vi "FR Make Default FRmeter settings.vi"() -> (3 "FFmeter settings":T1={"AC Source"={"AC Source type"=enum."Fluke 5XXX calibrator", "VISA"="", "Ref. clock (Hz)"=0.0, "status ref"=refnum}, "TWM pipe"="\\\\.\\pipe\\TWM:server", "Measurement status ref"=refnum, "TWM Status ref"=refnum, "Abort ref"=refnum, "DC meter"={"DC meter type"=enum."H/A/K 3458", "DC meter VISA"="", "NPLC"=10, "status ref"=refnum}, "Measurement properties"={"Measurement frequencies (Hz)"=[1000.0], "Sampling frequency (Hz)"=500000.0, "Signal amplitude (V)"=4.5, "AC-DC settle time (s)"=20.0, "Record length (multiples of period)"=[1000.0, 10000.0, 1000.0], "Measurement template file"=path "", "Row of START keyword"=1, "Row of STOP keyword"=0, "Calculate RMS from samples"=FALSE, "AC-DC warm up time (s)"=300.0, "Measurement template line"=[], "DC meter readings No."=10, "Algorithm"="TWM-WFFT", "Simultaneous measurement"=FALSE}, "Skip waiting ref"=refnum, "Octave paths"={"GNU Octave path"=path "C:/Program Files/GNU Octave/Octave-6.2.0/mingw64/bin", "TWM+QWTB path"=path "C:/Users/labina/Desktop/TWM-1.8.7.0-full/octprog", "lvlib path"=path "D:/martin/WAC/WACsw - github/control_software/Filter function meter/external libraries/GOLPI 0.7.3.1 source distribution LV 20.0 32 bit/lv_proc.dll"}, "Template definition"={"Keywords column"=0, "Sig. freq. column"=1, "Rec. len. column"=2, "Meas. points. row min to read"=9, "Meas. points. row max to read"=1509, "Properties column"=4, "Properties row start"=1, "Properties row end"=5, "Keyword START regexp"="", "Keyword STOP regexp"="", "HW data column"=7, "HW data row start"=1, "HW data row end"=3, "TIme and date column start"=3, "Digitizer value column start "=4, "DC mean column start "=6, "DC readings column start"=10}, "Recalculate-skip already calculated"=FALSE} {"Measurement properties"."Record length (multiples of period)" format="%#_3p"; "Measurement properties"."Sampling frequency (Hz)" format="%#_3p"; "Measurement properties"."Measurement frequencies (Hz)" format="%#_3p"})   [LabVIEW 2020]
doc: "Returns QPS set to default values."
uses:
  FR GUI/Type definitions/FFmeter settings.ctl
  General AC source/Type definitions/AC Source.ctl
  General AC source/Type definitions/AC Source type.ctl
  General DC meter/Type definitions/DC meter.ctl
  General DC meter/Type definitions/DC meter type.ctl
  FR Measurement/Type definitions/FR Measuement properties.ctl
  Type definitions/FR Template definition.ctl
  external libraries/varilib/varilib.lvlib
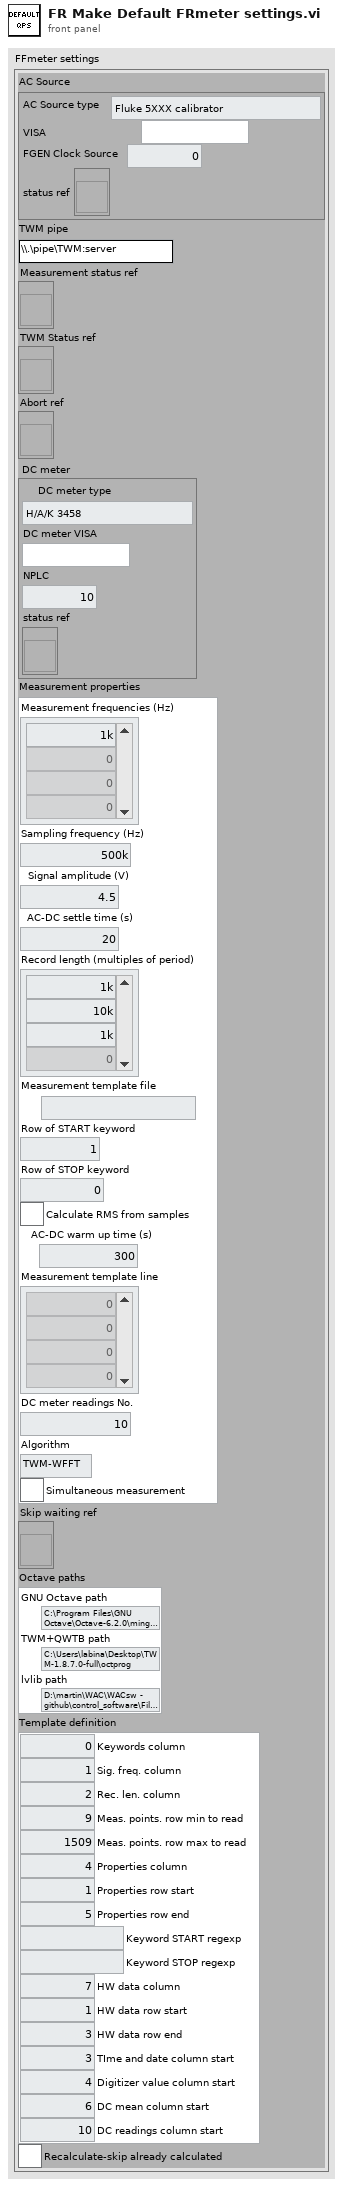
[diagram p1: front panel]
types:
  T1 = typedef "FFmeter settings.ctl" = cluster{"AC Source":T2, "TWM pipe":string, "Measurement status ref":refnum<vi>, "TWM Status ref":refnum<vi>, "Abort ref":refnum<vi>, "DC meter":T4, "Measurement properties":T6, "Skip waiting ref":refnum<vi>, "Octave paths":cluster{"GNU Octave path":path, "TWM+QWTB path":path, "lvlib path":path}, "Template definition":T7, "Recalculate-skip already calculated":bool}
  T2 = typedef "AC Source.ctl" = cluster{"AC Source type":T3, "VISA":refnum<visa-resource-name>, "Ref. clock (Hz)":dbl, "status ref":refnum<vi>}
  T3 = typedef "AC Source type.ctl" = enum16{"Fluke 5XXX calibrator", "Tektronix AFG3000 series", "dummy"}
  T4 = typedef "DC meter.ctl" = cluster{"DC meter type":T5, "DC meter VISA":refnum<visa-resource-name>, "NPLC":i32, "status ref":refnum<vi>}
  T5 = typedef "DC meter type.ctl" = enum16{"H/A/K 3458", "Fluke 8508A", "dummy", "Keithley 2182"}
  T6 = typedef "FR Measuement properties.ctl" = cluster{"Measurement frequencies (Hz)":dbl[], "Sampling frequency (Hz)":dbl, "Signal amplitude (V)":dbl, "AC-DC settle time (s)":dbl, "Record length (multiples of period)":dbl[], "Measurement template file":path, "Row of START keyword":i32, "Row of STOP keyword":i32, "Calculate RMS from samples":bool, "AC-DC warm up time (s)":dbl, "Measurement template line":i32[], "DC meter readings No.":i32, "Algorithm":string, "Simultaneous measurement":bool}
  T7 = typedef "FR Template definition.ctl" = cluster{"Keywords column":i32, "Sig. freq. column":i32, "Rec. len. column":i32, "Meas. points. row min to read":i32, "Meas. points. row max to read":i32, "Properties column":i32, "Properties row start":i32, "Properties row end":i32, "Keyword START regexp":string, "Keyword STOP regexp":string, "HW data column":i32, "HW data row start":i32, "HW data row end":i32, "TIme and date column start":i32, "Digitizer value column start ":i32, "DC mean column start ":i32, "DC readings column start":i32}
  T8 = cluster{"GNU Octave path":path, "TWM+QWTB path":path, "lvlib path":path}
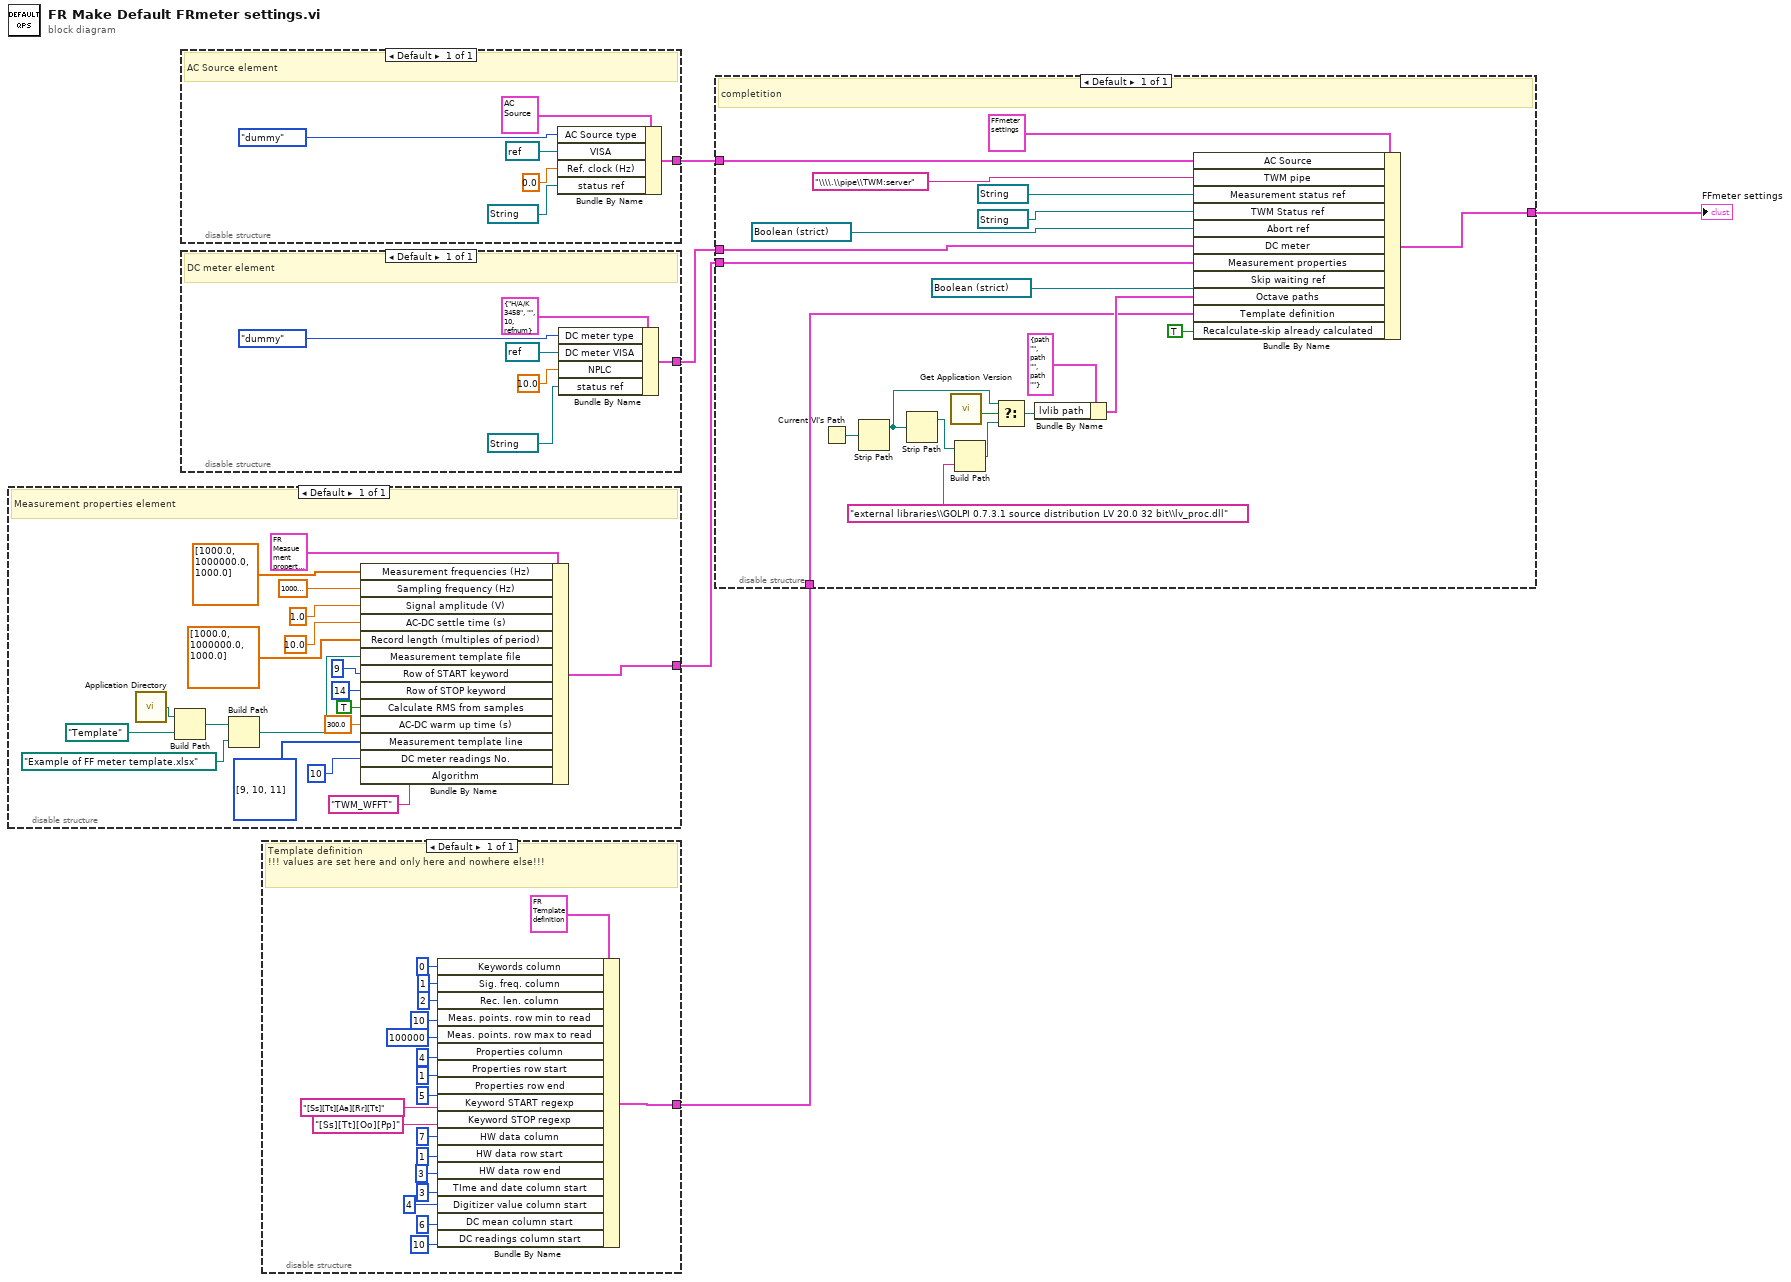
[diagram p0: block diagram]
diagram:
  n1 = disable-structure shown="Default" {
    disable-tunnel: [w23] -> w2
    frame Enabled {
      # "Measurement properties element"
      n2 = call <vilib>:"Application Directory.vi"() -> ("Application Directory"=w11:path)
      n3 = Build Path(base path=w11, name or relative path=path "Template") -> (appended path=w14:path)
      n4 = Build Path(base path=w14, name or relative path=path "Example of FF meter template.xlsx") -> (appended path=w12:path)
      n5 = Bundle By Name(cluster=T6 {"Measurement frequencies (Hz)"=[1000.0, 10000.0, 1000.0], "Sampling frequency (Hz)"=500000.0, "Signal amplitude (V)"=4.5, "AC-DC settle time (s)"=20.0, "Record length (multiples of period)"=[1000.0, 10000.0, 1000.0], "Measurement template file"=path "", "Row of START keyword"=0, "Row of STOP keyword"=0, "Calculate RMS from samples"=FALSE, "AC-DC warm up time (s)"=300.0, "Measurement template line"=[], "DC meter readings No."=10, "Algorithm"="TWM-WFFT", "Simultaneous measurement"=FALSE} ("Measurement properties"), "Measurement frequencies (Hz)"=dbl[] [1000.0, 1000000.0, 1000.0], "Sampling frequency (Hz)"=10000000.0, "Signal amplitude (V)"=1.0, "AC-DC settle time (s)"=10.0, "Record length (multiples of period)"=dbl[] [1000.0, 1000000.0, 1000.0], "Measurement template file"=w12, "Row of START keyword"=9, "Row of STOP keyword"=14, "Calculate RMS from samples"=TRUE, "AC-DC warm up time (s)"=300.0, "Measurement template line"=i32[] [9, 10, 11], "DC meter readings No."=10 ("No of readings"), "Algorithm"="TWM_WFFT") -> (w23:T6)
    }
  }
  n6 = disable-structure shown="Default" {
    disable-tunnel: [w29] -> w5
    frame Enabled {
      # "AC Source element"
      n7 = Bundle By Name(cluster=T2 {"AC Source type"=enum."Fluke 5XXX calibrator", "VISA"="", "Ref. clock (Hz)"=0.0, "status ref"=refnum} ("AC Source"), "AC Source type"=AC_Source_type."dummy" ("AWG type"), "VISA"=refnum<visa-resource-name> refnum, "Ref. clock (Hz)"=0.0, "status ref"=refnum<vi> refnum) -> (w29:T2)
    }
  }
  n8 = disable-structure shown="Default" {
    disable-tunnel: [w35] -> w3
    frame Enabled {
      # "DC meter element"
      n9 = Bundle By Name(cluster=T4 {"DC meter type"=enum."H/A/K 3458", "DC meter VISA"="", "NPLC"=10, "status ref"=refnum} ("DC meter"), "DC meter type"=DC_meter_type."dummy", "DC meter VISA"=refnum<visa-resource-name> refnum, "NPLC"=10.0, "status ref"=refnum<vi> refnum) -> (w35:T4)
    }
  }
  n10 = disable-structure shown="Default" {
    disable-tunnel: [w46] -> w1
    frame Enabled {
      # "Template definition\n!!! values are set here and only here and nowhere else!!!"
      n11 = Bundle By Name(cluster=T7 {"Keywords column"=0, "Sig. freq. column"=1, "Rec. len. column"=2, "Meas. points. row min to read"=9, "Meas. points. row max to read"=1509, "Properties column"=4, "Properties row start"=1, "Properties row end"=5, "Keyword START regexp"="[Ss][Tt][Aa][Rr][Tt]", "Keyword STOP regexp"="[Ss][Tt][Oo][Pp]", "HW data column"=7, "HW data row start"=1, "HW data row end"=3, "TIme and date column start"=3, "Digitizer value column start "=4, "DC mean column start "=6, "DC readings column start"=10} ("Template cells indexes"), "Keywords column"=0, "Sig. freq. column"=1, "Rec. len. column"=2, "Meas. points. row min to read"=10, "Meas. points. row max to read"=100000, "Properties column"=4, "Properties row start"=1, "Properties row end"=5, "Keyword START regexp"="[Ss][Tt][Aa][Rr][Tt]", "Keyword STOP regexp"="[Ss][Tt][Oo][Pp]", "HW data column"=7, "HW data row start"=1, "HW data row end"=3, "TIme and date column start"=3, "Digitizer value column start"=4, "DC mean column start"=6, "DC readings column start"=10) -> (w46:T7)
    }
  }
  n12 = disable-structure shown="Default" {
    disable-tunnel: [w76] -> w4
    disable-tunnel: w5 -> [w73]
    disable-tunnel: w3 -> [w69]
    disable-tunnel: w2 -> [w68]
    disable-tunnel: w1 -> [w57]
    frame Enabled {
      # "completition"
      n13 = Current VI's Path() -> (path=w65:path)
      n14 = Strip Path(path=w65) -> (stripped path=w64:path)  [unwired: 1 out]
      n15 = Strip Path(path=w64) -> (stripped path=w58:path)  [unwired: 1 out]
      n16 = call "Get Application Version.vi"() -> ("run time system"=w66:bool)  [unwired: 8 in, 3 out]
      n17 = Build Path(base path=w58, name or relative path="external libraries\\GOLPI 0.7.3.1 source distribution LV 20.0 32 bit\\lv_proc.dll") -> (appended path=w63:path)
      n18 = Select(t=w64, s=w66, f=w63) -> (s? t:f=w60:path)
      n19 = Bundle By Name(cluster=T8 {"GNU Octave path"=path "", "TWM+QWTB path"=path "", "lvlib path"=path ""} ("Octave paths"), "lvlib path"=w60) -> (w61:T8)
      n20 = Bundle By Name(cluster=T1 {"AC Source"={"AC Source type"=enum."Fluke 5XXX calibrator", "VISA"="", "Ref. clock (Hz)"=0.0, "status ref"=refnum}, "TWM pipe"="\\\\.\\pipe\\TWM:server", "Measurement status ref"=refnum, "TWM Status ref"=refnum, "Abort ref"=refnum, "DC meter"={"DC meter type"=enum."H/A/K 3458", "DC meter VISA"="", "NPLC"=10, "status ref"=refnum}, "Measurement properties"={"Measurement frequencies (Hz)"=[1000.0], "Sampling frequency (Hz)"=500000.0, "Signal amplitude (V)"=4.5, "AC-DC settle time (s)"=20.0, "Record length (multiples of period)"=[1000.0, 10000.0, 1000.0], "Measurement template file"=path "", "Row of START keyword"=1, "Row of STOP keyword"=0, "Calculate RMS from samples"=FALSE, "AC-DC warm up time (s)"=300.0, "Measurement template line"=[], "DC meter readings No."=10, "Algorithm"="TWM-WFFT", "Simultaneous measurement"=FALSE}, "Skip waiting ref"=refnum, "Octave paths"={"GNU Octave path"=path "C:/Program Files/GNU Octave/Octave-6.2.0/mingw64/bin", "TWM+QWTB path"=path "C:/Users/labina/Desktop/TWM-1.8.7.0-full/octprog", "lvlib path"=path "D:/martin/WAC/WACsw - github/control_software/Filter function meter/external libraries/GOLPI 0.7.3.1 source distribution LV 20.0 32 bit/lv_proc.dll"}, "Template definition"={"Keywords column"=0, "Sig. freq. column"=1, "Rec. len. column"=2, "Meas. points. row min to read"=9, "Meas. points. row max to read"=1509, "Properties column"=4, "Properties row start"=1, "Properties row end"=5, "Keyword START regexp"="", "Keyword STOP regexp"="", "HW data column"=7, "HW data row start"=1, "HW data row end"=3, "TIme and date column start"=3, "Digitizer value column start "=4, "DC mean column start "=6, "DC readings column start"=10}, "Recalculate-skip already calculated"=FALSE} ("FFmeter settings"), "AC Source"=w73, "TWM pipe"="\\\\.\\pipe\\TWM:server" ("TWM pipe name"), "Measurement status ref"=refnum<vi> refnum, "TWM Status ref"=refnum<vi> refnum, "Abort ref"=refnum<vi> refnum, "DC meter"=w69, "Measurement properties"=w68, "Skip waiting ref"=refnum<vi> refnum, "Octave paths"=w61, "Template definition"=w57, "Recalculate-skip already calculated"=TRUE ("skip calculated")) -> (w76:T1)
    }
  }
  "FFmeter settings" <- w4
